vi "Rebuild Local Report.vi"(9 "y":i32, 10 "UUT Result":T1, 11 "Station":i32) -> (3 "DetailTestResult":string[][](array[string]))   [LabVIEW 2019, in "Full User Interface.lvlib"]
uses:
  Full User Interface.lvlib
  Test Unit/UUT Result.ctl
  <vilib>/Test Bench Framework/Test Executive.lvlibp/TestEngine/TestEngine/TestEngine/Typedefs/Report General.ctl
  <vilib>/Utility/miscctls.llb/LVMapReplaceAction.ctl
  <vilib>/Test Bench Framework/Test Executive.lvlibp/TestEngine/TestEngine/TestEngine/Test Engine.lvclass
  Test Unit/Test Unit.lvlib
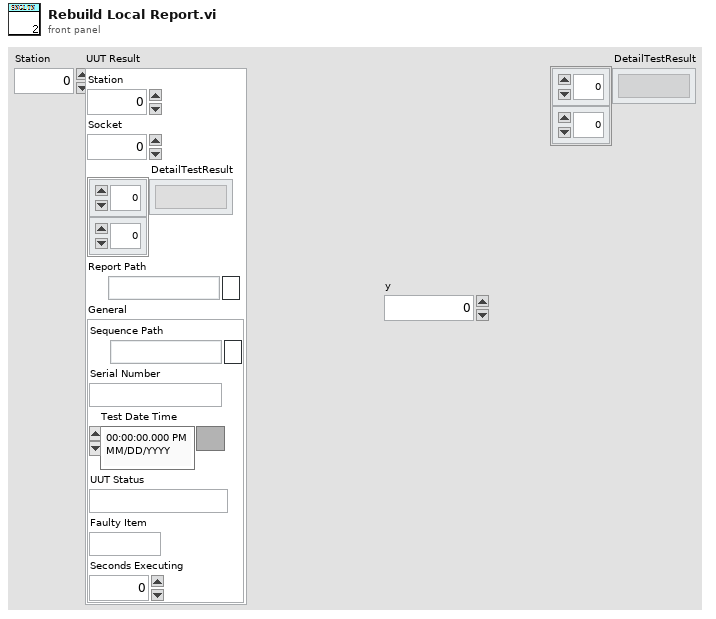
[diagram p1: front panel]
types:
  T1 = typedef "Test Unit.lvlib/UUT Result.ctl" = cluster{"Station":i32, "Socket":i32, "DetailTestResult":string[][], "Report Path":path, "General":T2}
  T2 = typedef "Test Executive.lvlibp/Test Engine.lvlib/Test Engine.lvclass/Report General.ctl" = cluster{"Sequence Path":path, "Serial Number":string, "Test Date Time":timestamp, "UUT Status":string, "Faulty Item":string, "Seconds Executing":dbl}
  T3 = typedef "LVMapReplaceAction.ctl" = enum32{"Modify Entry only if found", "Add or Modify Entry", "Delete Entry"}
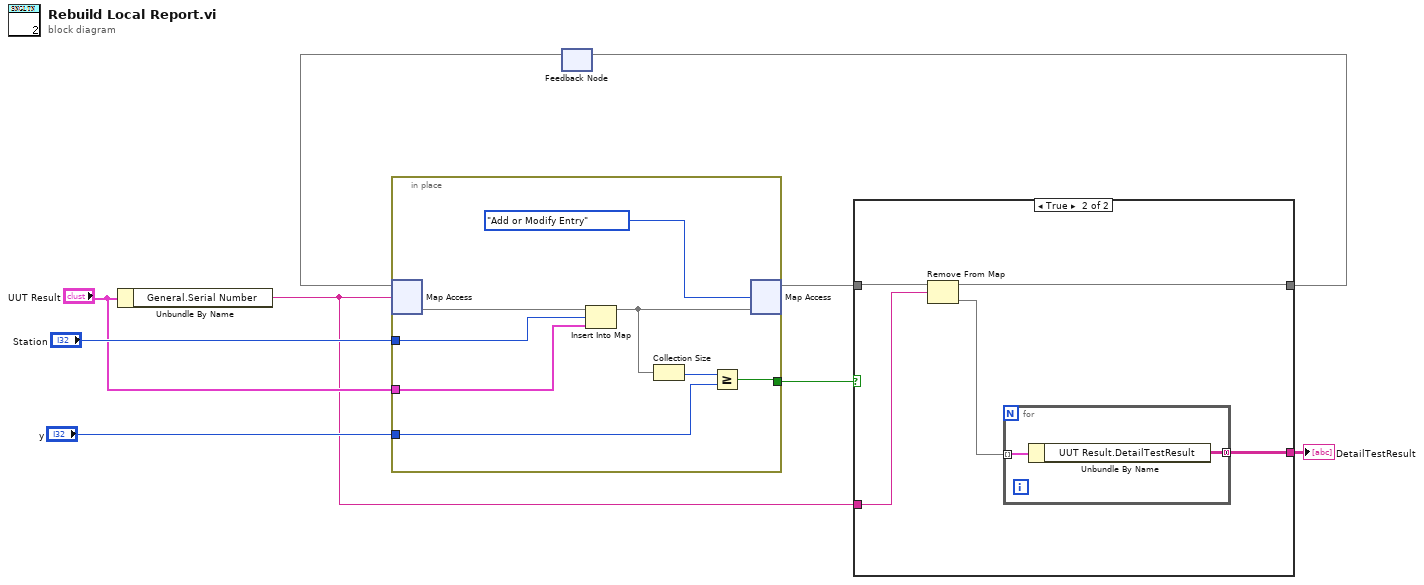
[diagram p0: block diagram]
diagram:
  n1 = Unbundle By Name("UUT Result") -> ("General.Serial Number"=w2:string)
  n2 = feedback #1() -> (w9:map{string, map{i32, T1}})  [unwired: 1 in]
  n3 = in-place {
    in-place-border: "Station" -> [w15]
    in-place-border: "UUT Result" -> [w14]
    in-place-border: "y" -> [w11]
    in-place-border: [w10] -> w5
    n4 = in-place-map #2(w9, w2) -> (w16:map{i32, T1})  [unwired: 1 in, 1 out]
    n5 = Insert Into Map(map in=w16, key=w15, value=w14) -> (map out=w13:map{i32, T1})  [unwired: 2 out]
    n6 = Collection Size(1:w13) -> (0:w12:i32)
    n7 = Greater Or Equal?(x=w12, y=w11) -> (x >= y?=w10:bool)
    n8 = in-place-map #2(w13, LVMapReplaceAction."Add or Modify Entry" ("action")) -> (w4:map{string, map{i32, T1}})  [unwired: 2 out]
  }
  n9 = case shown="True" w5 {
    tunnel: w4 -> [w18 w23]
    tunnel: [w18 w22] -> w3
    tunnel: w2 -> [_ w21]
    tunnel: [_ w19] -> w1
    frame False {
    }
    frame True {
      n10 = Remove From Map(10:w21, 11:w23) -> (1:w20:map{i32, T1}, 3:w22:map{string, map{i32, T1}})  [unwired: 1 out]
      n11 = for {
        tunnel: w20 -> [w25] mode=indexing
        tunnel: [w24] -> w19 mode=concatenating
        n12 = Unbundle By Name(w25) -> ("UUT Result.DetailTestResult"=w24:string[][])
      }
    }
  }
  "DetailTestResult" <- w1
  n13 = feedback-in #1(w3) -> ()
